vi "Expand Greyscale Image Data.vi"(0 "Greyscale Data":u8[][](array[numeric]), 1 "Factor":u16=2) -> (2 "Expanded Greyscale Data":u8[][](array[numeric]))   [LabVIEW 2020, in "image.lvlib"]
doc: "Expand the greyscale image data by the specified scale factor."
uses:
  image.lvlib
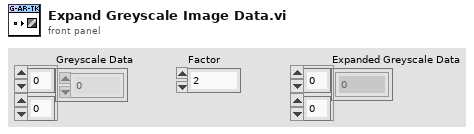
[diagram p1: front panel]
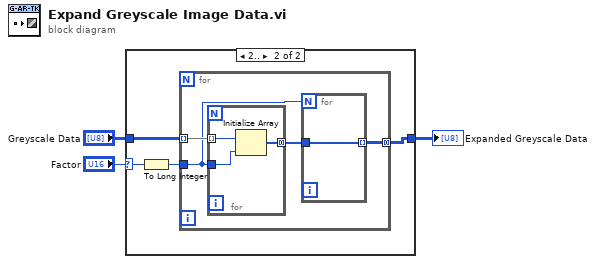
[diagram p0: block diagram]
diagram:
  n1 = case shown="2.." "Factor" {
    selector: "Factor" -> [_ w8]
    tunnel: "Greyscale Data" -> [w4 w7]
    tunnel: [w4 w6] -> w1
    frame Default {
    }
    frame 2.. {
      n2 = To Long Integer(number=w8) -> (32bit integer=w5:i32)
      n3 = for {
        tunnel: w7 -> [w12] mode=indexing
        tunnel: [w10] -> w6 mode=concatenating
        tunnel: w5 -> [w9]
        n4 = for {
          tunnel: w12 -> [w16] mode=indexing
          tunnel: w9 -> [w15]
          tunnel: [w14] -> w11 mode=concatenating
          n5 = Initialize Array(w16, w15) -> (w14:u8[])
        }
        n6 = for {
          N: w9 -> [_]
          tunnel: w11 -> [w13]
          tunnel: [w13] -> w10 mode=indexing
        }
      }
    }
  }
  "Expanded Greyscale Data" <- w1
